vi "檢測_距離_VI.vi"(8 "error in (no error)":errorcluster, 9 "找圓":cluster{"X":sgl, "Y":sgl}[](array[cluster]), 10 "找邊":cluster{"X":sgl, "Y":sgl}[](array[cluster]), 11 "Image":T1) -> (0 "error out":errorcluster, 1 "Distances":sgl[][](array[numeric]), 2 "min value":sgl, 3 "Image Out":T1)   [LabVIEW 2015]
uses:
  <vilib>/vision/Image Controls.llb/IMAQ Image.ctl
  <vilib>/vision/NI_Vision_Development_Module.lvlib
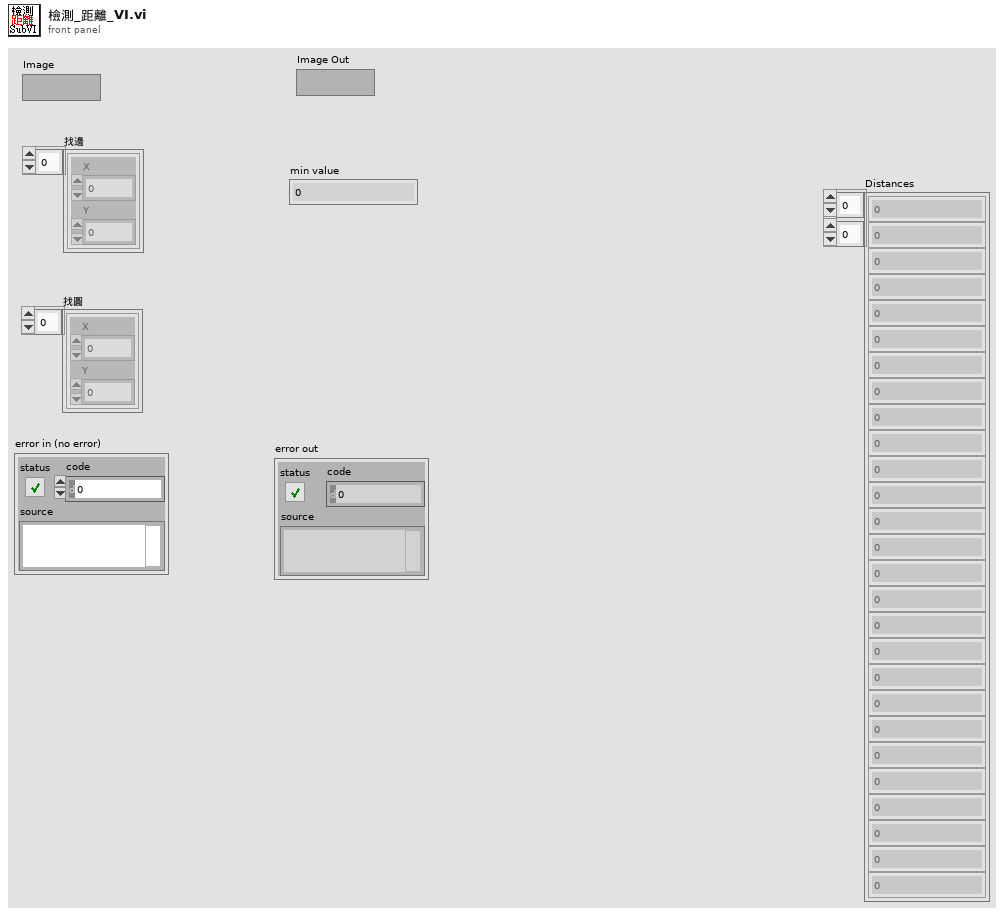
[diagram p1: front panel]
types:
  T1 = typedef "IMAQ Image.ctl" = refnum<image>
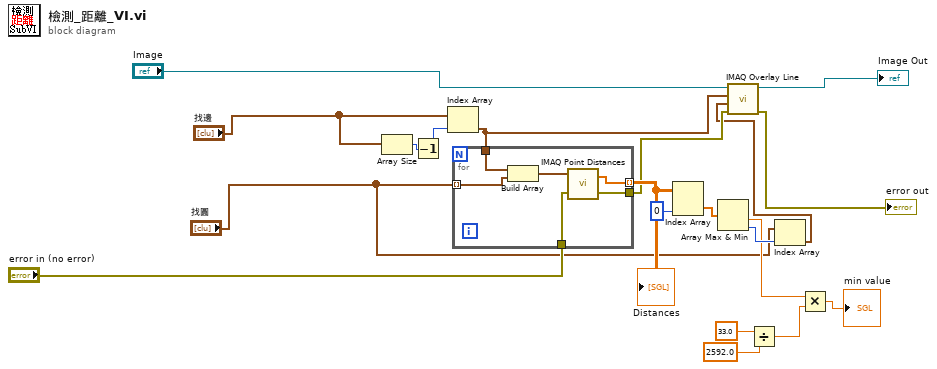
[diagram p0: block diagram]
diagram:
  n1 = Array Size(array="找邊") -> (size(s)=w10:i32)
  n2 = Decrement(x=w10) -> (x-1=w9:i32)
  n3 = Index Array(array="找邊", index=w9) -> (element=w20:cluster{"X":sgl, "Y":sgl})
  n4 = for {
    tunnel: "找圓" -> [w25] mode=indexing
    tunnel: w20 -> [w26]
    tunnel: [w23] -> w17 mode=indexing
    tunnel: "error in (no error)" -> [w22]
    tunnel: [w21] -> w4
    n5 = Build Array(w26, w25) -> (w24:cluster{"X":sgl, "Y":sgl}[])
    n6 = call "IMAQ Point Distances"("Points"=w24, "error in (no error)"=w22) -> ("Distances"=w23:sgl[], "error out"=w21:errorcluster)  [unwired: 3 in]
  }
  "Distances" <- w17
  n7 = Index Array(array=w17, index (col)=0 ("disabled index (col)")) -> (element=w19:sgl[])  [unwired: 1 in]
  n8 = Array Max & Min(array=w19) -> (min value=w15:sgl, min index (indices)=w18:i32)  [unwired: 2 out]
  n9 = Divide(x=33.0, y=2592.0) -> (x/y=w14:dbl)
  n10 = Index Array(array="找圓", index=w18) -> (element=w1:cluster{"X":sgl, "Y":sgl})
  n11 = call "IMAQ Overlay Line"("error in (no error)"=w4, "End Point"=w1, "Start Point"=w20, "Image"="Image") -> ("error out"=→"error out":errorcluster, "Image Out"=→"Image Out":T1)  [unwired: 6 in]
  n12 = Multiply(x=w15, y=w14) -> (x*y=→"min value":dbl)
